vi "Leitor_corrente_sub1.vi"(0 "Numeric":dbl format="%#_13g") -> (4 "max value":dbl)   [LabVIEW 2016]
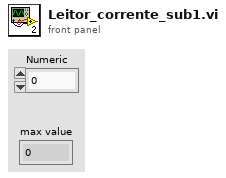
[diagram p1: front panel]
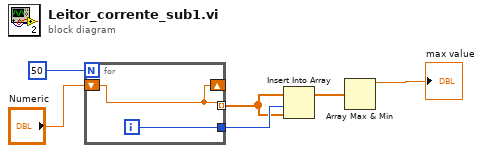
[diagram p0: block diagram]
diagram:
  n1 = for {
    N: 50 -> [_]
    tunnel: [w7] -> w5 mode=indexing
    tunnel: [w8] -> w6
    shift-right: [w7] -> _
    shift-left: "Numeric" -> [w7]
    i -> [w8]
  }
  n2 = Insert Into Array(array=w5, index=w6, new element=w5) -> (w2:dbl[])
  n3 = Array Max & Min(array=w2) -> (max value=→"max value":dbl)  [unwired: 3 out]
